vi "SetOutputCurrent.vi"(8 "error in (no error)":errorcluster, 10 "Current":dbl, 11 "RMX4120 in":refnum<class "RMX4120.lvclass">) -> (0 "error out":errorcluster, 3 "RMX4120 out":refnum<class "RMX4120.lvclass">)   [LabVIEW 2023, in "RMX4120.lvclass"]
uses:
  RMX4120.lvclass
  RMX4120.lvclass/RMX4120.ctl
  RMXPowerSupply.lvclass
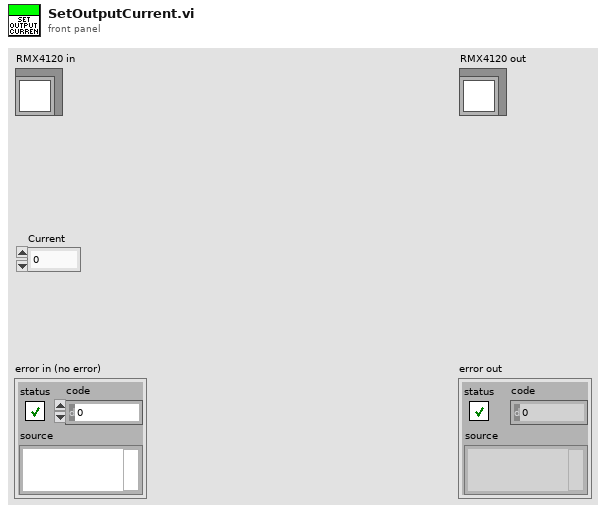
[diagram p1: front panel]
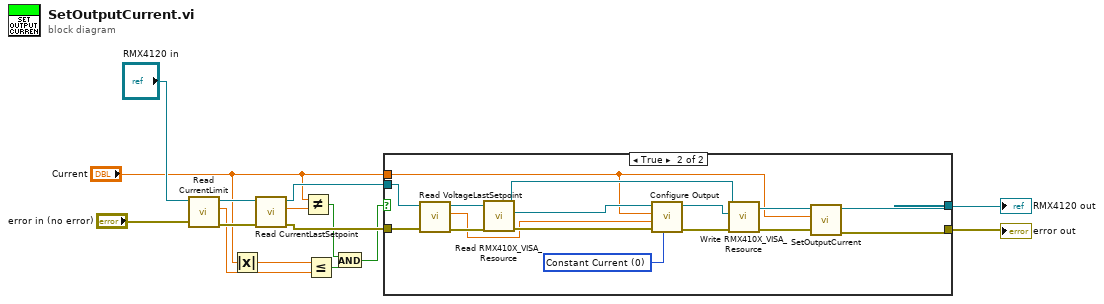
[diagram p0: block diagram]
diagram:
  n1 = call-dynamic "Read CurrentLimit.vi"("error in (no error)"="error in (no error)", "RMXPowerSupply in"="RMX4120 in") -> ("error out"=w7:errorcluster, "CurrentLimit"=w4:dbl, "RMXPowerSupply out"=w8:refnum<class "RMX4120.lvclass">)  [unwired: 7 in]
  n2 = Absolute Value(x="Current") -> (abs(x)=w5:dbl)
  n3 = call-dynamic "Read CurrentLastSetpoint.vi"("error in (no error)"=w7, "RMXPowerSupply in"=w8) -> ("error out"=w14:errorcluster, "CurrentLastSetpoint"=w15:dbl, "RMXPowerSupply out"=w13:refnum<class "RMX4120.lvclass">)  [unwired: 7 in]
  n4 = Not Equal?(x="Current", y=w15) -> (x != y?=w2:bool)
  n5 = Less Or Equal?(x=w5, y=w4) -> (x <= y?=w3:bool)
  n6 = And(x=w2, y=w3) -> (x .and. y?=w1:bool)
  n7 = case shown="True" w1 {
    tunnel: w14 -> [w17 w27]
    tunnel: w13 -> [w16 w24]
    tunnel: "Current" -> [_ w18]
    tunnel: [w17 w19] -> w12
    tunnel: [w16 w20] -> w11
    frame False {
    }
    frame True {
      w30 = 0 items=["Constant Current", "Constant Voltage"] ("Operation Mode (0: Constant Current)")
      n8 = call-dynamic "Read VoltageLastSetpoint.vi"("error in (no error)"=w27, "RMXPowerSupply in"=w24) -> ("error out"=w26:errorcluster, "VoltageLastSetpoint"=w23:dbl, "RMXPowerSupply out"=w25:refnum<class "RMX4120.lvclass">)  [unwired: 7 in]
      n9 = call-dynamic "Read RMX410X_VISA_Resource.vi"("error in (no error)"=w26, "RMXPowerSupply in"=w25) -> ("error out"=w33:errorcluster, "RMX410X_VISA_Resource"=w31:refnum<visa-resource-name>, "RMXPowerSupply out"=w28:refnum<class "RMX4120.lvclass">)  [unwired: 7 in]
      n10 = call "Configure Output.vi"("Operation Mode (0: Constant Current)"=w30, "error in (no error)"=w33, "Output Voltage (0 V)"=w23, "Output Current (0 A)"=w18, "VISA resource name"=w31) -> ("error out"=w32:errorcluster, "VISA resource name out"=w29:refnum<visa-resource-name>)  [unwired: 5 in]
      n11 = call-dynamic "Write RMX410X_VISA_Resource.vi"("error in (no error)"=w32, "RMX410X_VISA_Resource"=w29, "RMXPowerSupply in"=w28) -> ("error out"=w21:errorcluster, "RMXPowerSupply out"=w22:refnum<class "RMX4120.lvclass">)  [unwired: 7 in]
      n12 = call-parent "SetOutputCurrent.vi"("error in (no error)"=w21, "Current"=w18, "RMXPowerSupply in"=w22) -> ("error out"=w19:errorcluster, "RMXPowerSupply out"=w20:refnum<class "RMX4120.lvclass">)  [unwired: 7 in]
    }
  }
  "error out" <- w12
  "RMX4120 out" <- w11
